vi "forward+backward.vi"(8 "Robot angle":dbl, 9 "Actual robot location":dbl[](array[numeric]), 10 "wait time (ms)":dbl, 11 "Forward/backward":string) -> (3 "New robot location":dbl[](array[numeric]))   [LabVIEW 2015]
uses:
  <vilib>/myRIO/Instrument Drivers/Onboard IO/PWM/typedefs/PWM Reference.ctl
  <vilib>/myRIO/Common/Instrument Driver Framework/Utilities/typedefs/myRIO Generic Hardware Reference.ctl
  <vilib>/myRIO/Common/Instrument Driver Framework/Utilities/typedefs/Hardware Version Enum.ctl
  <vilib>/myRIO/Common/Instrument Driver Framework/Utilities/typedefs/myRIO v1.0 Reference.ctl
  <vilib>/myRIO/Common/Instrument Driver Framework/Utilities/typedefs/Generic FPGA Reference.ctl
  <vilib>/myRIO/Common/Instrument Driver Framework/myRIO v1.0/PWM/typedefs/PWM Channels Enum.ctl
  <vilib>/myRIO/Instrument Drivers/Onboard IO/PWM/typedefs/PWM Configuration.ctl
  <vilib>/userdefined/High Color/nirio_resource_hc.ctl
  <vilib>/myRIO/Common/Instrument Driver Framework/Utilities/vis/Is FPGA Ref Available.vi
  <vilib>/myRIO/Common/Instrument Driver Framework/myRIO v1.0/PWM/vis/myRIO v1.1 Open PWM.vi
  <vilib>/myRIO/Instrument Drivers/Onboard IO/PWM/vis/Set Duty Cycle and Frequency.vi
  <vilib>/myRIO/Common/Instrument Driver Framework/Utilities/vis/Validate Channels.vi
  <vilib>/myRIO/Common/Instrument Driver Framework/myRIO v1.0/PWM/vis/myRIO v1.0 Reserve PWM.vi
  <vilib>/myRIO/Common/Instrument Driver Framework/myRIO v1.0/PWM/vis/myRIO v1.0 Build MUX Configuration PWM.vi
  <vilib>/myRIO/Common/Instrument Driver Framework/myRIO v1.0/Resource Manager/vis/myRIO v1.0 Reserve Channel List.vi
  <vilib>/myRIO/Common/Instrument Driver Framework/myRIO v1.0/Resource Manager/vis/myRIO v1.0 Create Configuration List.vi
  <vilib>/myRIO/Common/Instrument Driver Framework/myRIO v1.0/Resource Manager/vis/myRIO v1.0 Reserve Channel.vi
  <vilib>/myRIO/Common/Instrument Driver Framework/myRIO v1.0/Resource Manager/vis/myRIO v1.0 Unreserve Channel.vi
  <vilib>/myRIO/Common/Instrument Driver Framework/myRIO v1.0/Resource Manager/vis/myRIO v1.0 Build Mutex Name.vi
  <vilib>/Utility/VariantDataType/GetNumericInfo.vi
  <vilib>/Utility/error.llb/Error Cluster From Error Code.vi
  <vilib>/myRIO/Common/Instrument Driver Framework/myRIO v1.0/myRIO v1.1 Open.vi
  <vilib>/myRIO/Common/Instrument Driver Framework/Utilities/vis/IO Manager.vi
  <vilib>/myRIO/Common/Instrument Driver Framework/Utilities/vis/Configuration Manager.vi
  <vilib>/myRIO/Common/Instrument Driver Framework/myRIO v1.0/Resource Manager/vis/myRIO v1.0 Configure IO.vi
  <vilib>/myRIO/Common/Instrument Driver Framework/myRIO v1.0/myRIO v1.0 Close.vi
  <vilib>/myRIO/Common/Instrument Driver Framework/myRIO v1.0/PWM/vis/myRIO v1.0 Write PWM.vi
  <vilib>/myRIO/Express VI/Onboard IO/PWM/PWM Express VI.xnode
  <vilib>/myRIO/Instrument Drivers/Onboard IO/PWM/vis/myRIO PWM Open.xnode
  <vilib>/myRIO/Instrument Drivers/Onboard IO/PWM/PWM.lvlib
panel:
  out "End distance":dbl
  out "Start distance":dbl
  out "error out 2":errorcluster
  out "error out":errorcluster
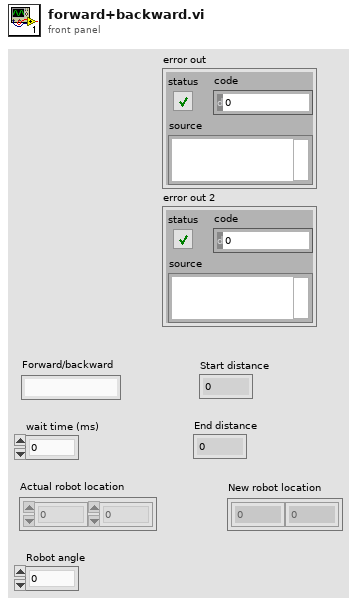
[diagram p1: front panel]
types:
  T1 = typedef "PWM.lvlib/PWM Reference.ctl" = cluster{"myRIO Reference":T2, "PWM Channels Enum":T6, "PWM Configuration":T7}
  T2 = typedef "myRIO Generic Hardware Reference.ctl" = cluster{"myRIO Model":T3, "myRIO Hardware Reference":T4}
  T3 = typedef "Hardware Version Enum.ctl" = enum16{"Unknown", "myRIO-1900", "myRIO-1950", "roboRIO"}
  T4 = typedef "myRIO v1.0 Reference.ctl" = cluster{"Generic FPGA Reference":T5, "Allow multiple opens":bool}
  T5 = typedef "Generic FPGA Reference.ctl" = refnum<k20>
  T6 = typedef "PWM Channels Enum.ctl" = enum16{"Not Connected", "C/PWM0", "C/PWM1", "A/PWM0", "A/PWM1", "A/PWM2", "B/PWM0", "B/PWM1", "B/PWM2", "PWM/PWM0", "PWM/PWM1", "PWM/PWM2", "PWM/PWM3", "PWM/PWM4", "PWM/PWM5", "PWM/PWM6", "PWM/PWM7", "PWM/PWM8", "PWM/PWM9"}
  T7 = typedef "PWM.lvlib/PWM Configuration.ctl" = cluster{"Frequency":dbl, "Duty Cycle":dbl}
  T8 = typedef "nirio_resource_hc.ctl" = tag
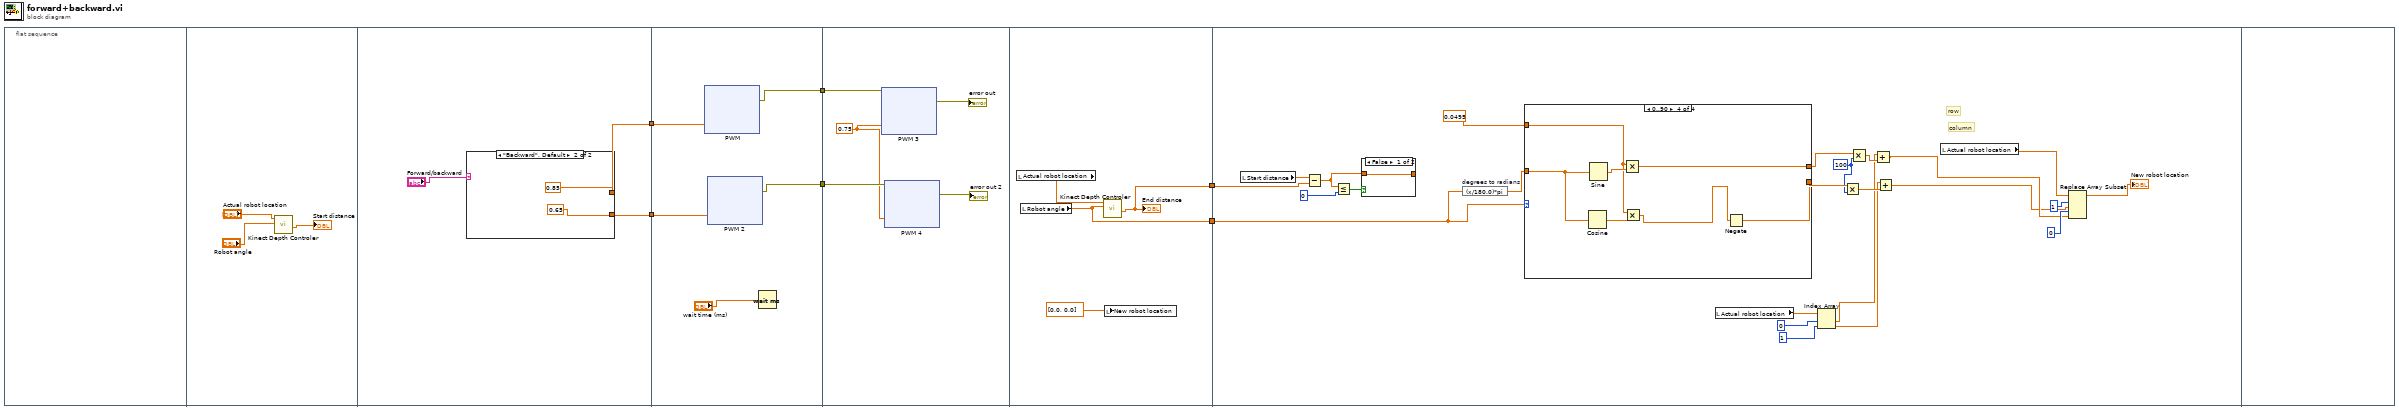
[diagram p0: block diagram]
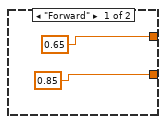
[diagram p2: hidden frame]
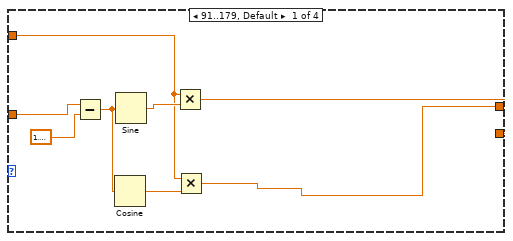
[diagram p3: hidden frame]
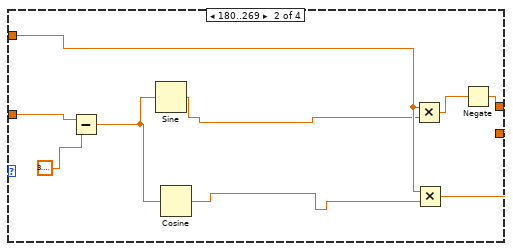
[diagram p4: hidden frame]
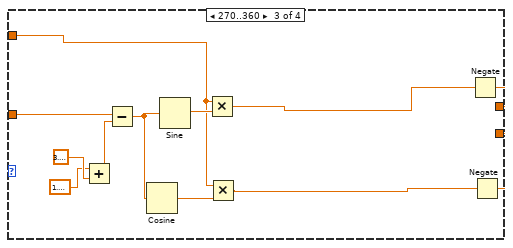
[diagram p5: hidden frame]
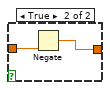
[diagram p6: hidden frame]
diagram:
  n1 = flat-sequence {
    tunnel: [w11] -> w6
    tunnel: [w10] -> w5
    tunnel: w6 -> [w20]
    tunnel: w5 -> [w19]
    tunnel: [w18] -> w4
    tunnel: [w17] -> w3
    tunnel: w4 -> [w96]
    tunnel: w3 -> [w95]
    tunnel: [w169] -> w2
    tunnel: [w168] -> w1
    tunnel: w2 -> [w193]
    tunnel: w1 -> [w184]
    frame #0 {
    }
    frame #1 {
      n2 = call "Kinect Depth Controler.vi"("Angle"="Robot angle", "Robot Location"="Actual robot location") -> ("Closest distance"=→"Start distance":dbl)  [unwired: 7 in, 2 out]
    }
    frame #2 {
      n3 = case shown="\"Backward\", Default" "Forward/backward" {
        tunnel: [0.65 0.85] -> w11
        tunnel: [0.85 0.65] -> w10
        frame "Forward" {
        }
        frame "Backward", Default {
        }
      }
    }
    frame #3 {
      n4 = xnode "PWM"("Duty Cycle"=w20) -> ("error out"=w18:errorcluster)  [unwired: 1 in]
      n5 = xnode "PWM 2"("Duty Cycle"=w19) -> ("error out"=w17:errorcluster)  [unwired: 1 in]
      n6 = Wait (ms)(milliseconds to wait="wait time (ms)") -> ()  [unwired: 1 out]
    }
    frame #4 {
      w92 = 0.75
      n7 = xnode "PWM 3"("Duty Cycle"=w92, "error in (no error)"=w96) -> ("error out"=→"error out":errorcluster)
      n8 = xnode "PWM 4"("Duty Cycle"=w92, "error in (no error)"=w95) -> ("error out"=→"error out 2":errorcluster)
    }
    frame #5 {
      n9 = local read "Actual robot location"() -> (w170:dbl[])
      n10 = local read "Robot angle"() -> (w168:dbl)
      n11 = call "Kinect Depth Controler.vi"("Angle"=w168, "Robot Location"=w170) -> ("Closest distance"=w169:dbl)  [unwired: 7 in, 2 out]
      "End distance" <- w169
      n12 = local write "New robot location"(dbl[] [0.0, 0.0] ("New robot location")) -> ()
    }
    frame #6 {
      w189 = 100
      # "column"
      # "row"
      n13 = local read "Start distance"() -> (w194:dbl)
      n14 = Subtract(x=w194, y=w193) -> (x-y=w191:dbl)
      n15 = Less Or Equal?(x=w191, y=0) -> (x <= y?=w192:bool)
      n16 = case shown="False" w192 {
        tunnel: w191 -> [w230 w232]
        tunnel: [w230 w231] -> _
        frame False {
        }
        frame True {
          n17 = Negate(x=w232) -> (-x=w231:dbl)
        }
      }
      n18 = expression code="(x/180.0)*pi" "degrees to radians"(w184) -> (w188:dbl)
      n19 = case shown="0..90" w184 {
        tunnel: w188 -> [w198 w209 w219 w229]
        tunnel: 0.0495 -> [w200 w210 w218 w227]
        tunnel: [w195 w207 w211 w226] -> w187
        tunnel: [w196 w206 w212 w224] -> w190
        frame 91..179, Default {
          n20 = Subtract(x=w198, y=1.5707963267948966) -> (x-y=w199:dbl)
          n21 = Cosine(x=w199) -> (cos(x)=w201:dbl)
          n22 = Sine(x=w199) -> (sin(x)=w202:dbl)
          n23 = Multiply(x=w200, y=w202) -> (x*y=w196:dbl)
          n24 = Multiply(x=w200, y=w201) -> (x*y=w195:dbl)
        }
        frame 180..269 {
          n25 = Subtract(x=w209, y=3.141592653589793) -> (x-y=w205:dbl)
          n26 = Sine(x=w205) -> ()  [unwired: 1 out]
          n27 = Cosine(x=w205) -> (cos(x)=w204:dbl)
          n28 = Multiply(x=w210, y=w205) -> (x*y=w208:dbl)
          n29 = Multiply(x=w210, y=w204) -> (x*y=w206:dbl)
          n30 = Negate(x=w208) -> (-x=w207:dbl)
        }
        frame 270..360 {
          n31 = Add(x=1.5707963267948966, y=3.141592653589793) -> (x+y=w213:dbl)
          n32 = Subtract(x=w219, y=w213) -> (x-y=w222:dbl)
          n33 = Cosine(x=w222) -> (cos(x)=w221:dbl)
          n34 = Sine(x=w222) -> (sin(x)=w220:dbl)
          n35 = Multiply(x=w218, y=w220) -> (x*y=w216:dbl)
          n36 = Multiply(x=w218, y=w221) -> (x*y=w217:dbl)
          n37 = Negate(x=w216) -> (-x=w212:dbl)
          n38 = Negate(x=w217) -> (-x=w211:dbl)
        }
        frame 0..90 {
          n39 = Cosine(x=w229) -> (cos(x)=w223:dbl)
          n40 = Sine(x=w229) -> (sin(x)=w228:dbl)
          n41 = Multiply(x=w227, y=w228) -> (x*y=w226:dbl)
          n42 = Multiply(x=w227, y=w223) -> (x*y=w225:dbl)
          n43 = Negate(x=w225) -> (-x=w224:dbl)
        }
      }
      n44 = local read "Actual robot location"() -> (w183:dbl[])
      n45 = Index Array(array=w183, index #1=0, index #2=1) -> (element #1=w179:dbl, element #2=w180:dbl)
      n46 = Multiply(x=w190, y=w189) -> (x*y=w185:dbl)
      n47 = Multiply(x=w187, y=w189) -> (x*y=w186:dbl)
      n48 = Add(x=w179, y=w186) -> (x+y=w173:dbl)
      n49 = Add(x=w180, y=w185) -> (x+y=w172:dbl)
      n50 = local read "Actual robot location"() -> (w178:dbl[])
      n51 = Replace Array Subset(array=w178, new element #1=w172, index #1=1, new element #2=w173, index #2=0) -> (→"New robot location":dbl[])
    }
    frame #7 {
    }
  }
